vi "SpectrumBinning_NoGraph.vi"(3 "XScale.Maximum":dbl, 4 "BinType":T1, 5 "BinWidth":dbl=1.0, 7 "Enable":bool=TRUE, 8 "error in (no error)":errorcluster, 9 "Signal":dbl[](array[numeric]), 10 "m/z Array":dbl[](array[numeric]), 11 "XScale.Minimum":dbl) -> (0 "error out":errorcluster, 1 "Spectrum":dbl[](array[numeric]), 2 "m/z Array":dbl[](array[numeric]))   [LabVIEW 2013]
uses:
  BinType.ctl
  <vilib>/Analysis/baseanly.llb/Mean (DBL).vi
  <vilib>/Analysis/NI_AALBase.lvlib
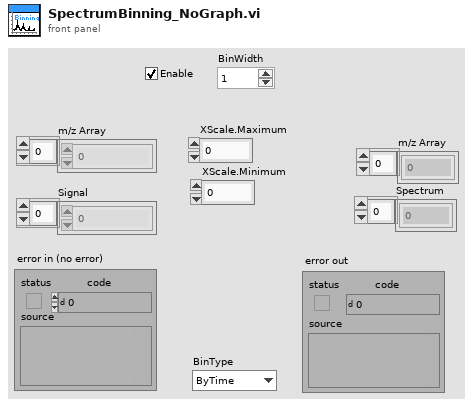
[diagram p1: front panel]
types:
  T1 = typedef "BinType.ctl" = enum16{"ByTime", "ByScreen", "ByMass", "ToUnitMass"}
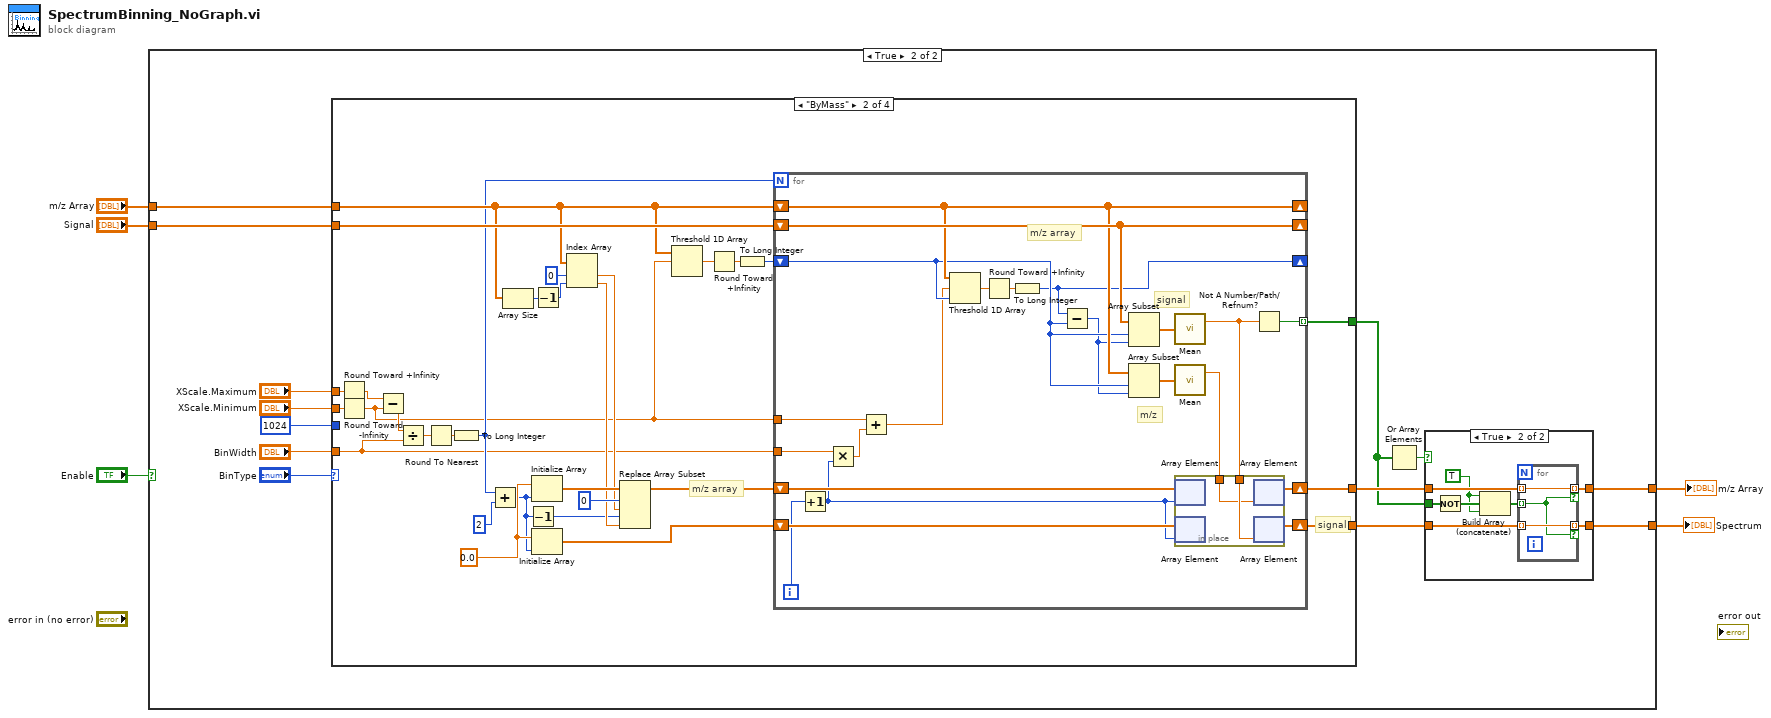
[diagram p0: block diagram]
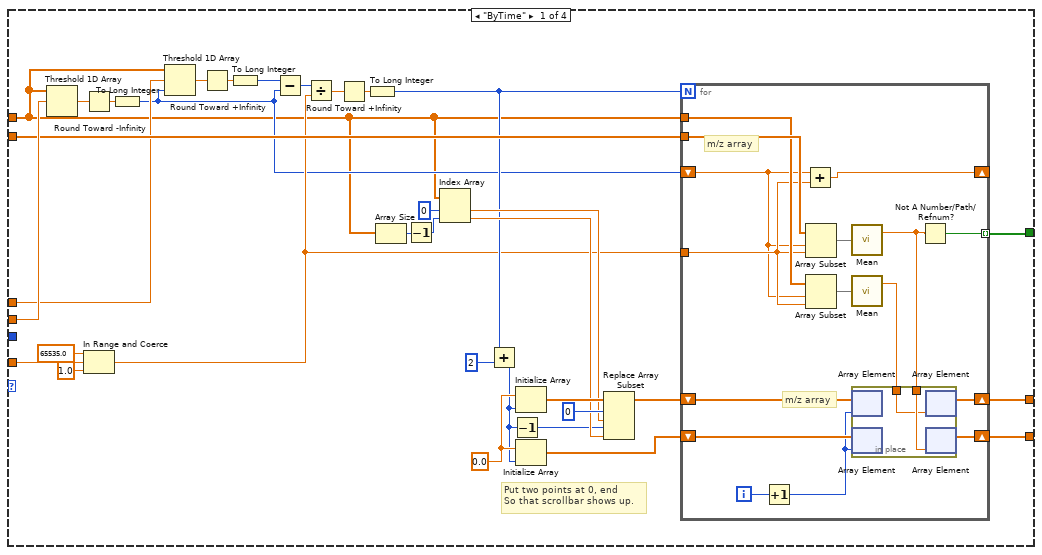
[diagram p4: hidden frame]
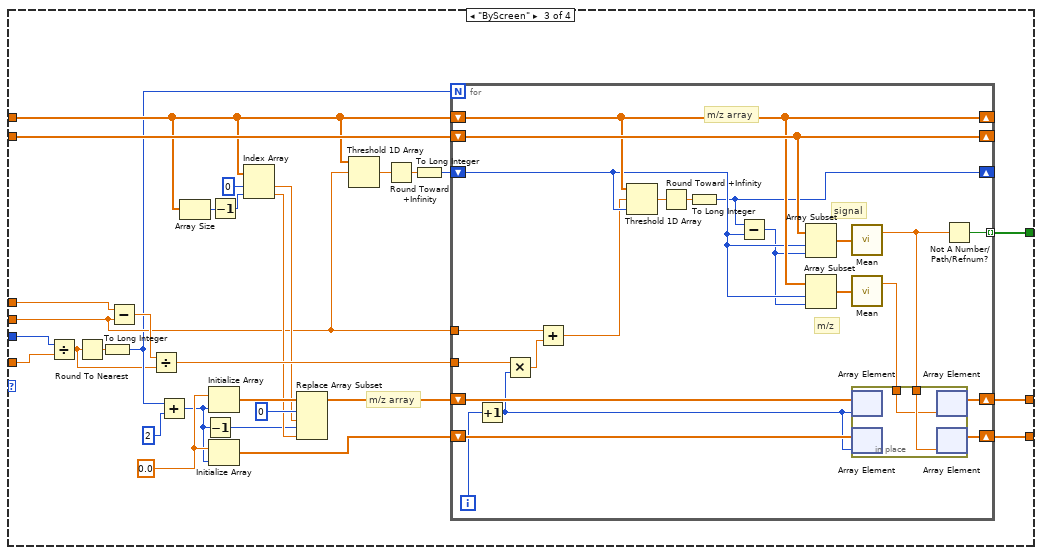
[diagram p5: hidden frame]
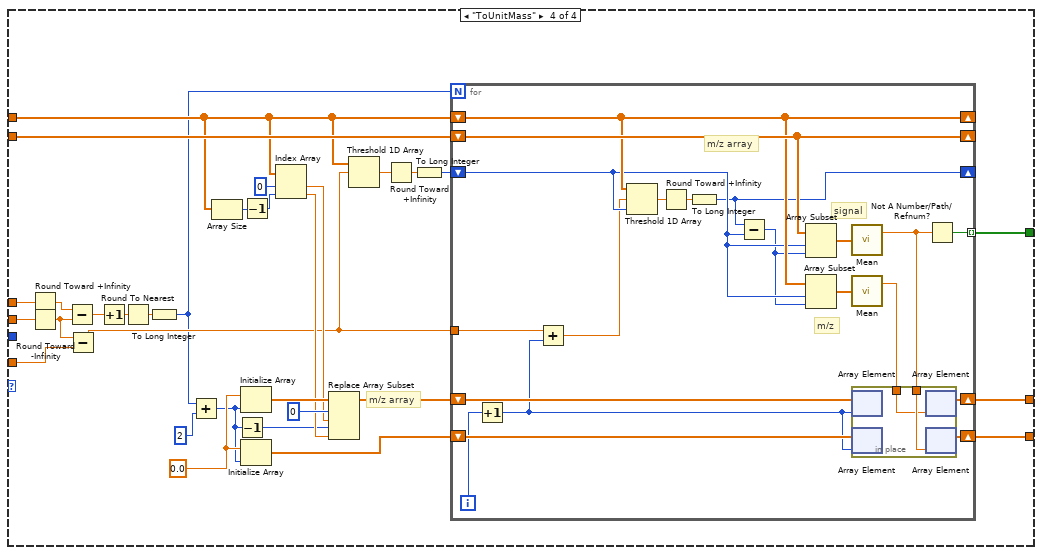
[diagram p6: hidden frame]
diagram:
  n1 = case shown="True" "Enable" {
    tunnel: "Signal" -> [w7 w14]
    tunnel: "m/z Array" -> [w6 w13]
    tunnel: [w6 w9] -> w2
    tunnel: [w7 w8] -> w1
    frame False {
    }
    frame True {
      n2 = case shown="\"ByMass\"" "BinType" {
        tunnel: w14 -> [w53 w115 w169 w224]
        tunnel: w13 -> [w34 w106 w158 w215]
        tunnel: "XScale.Maximum" -> [w38 w100 w152 w209]
        tunnel: "XScale.Minimum" -> [w54 w96 w148 w205]
        tunnel: u32 1024 ("Width") -> [_ _ w145 _]
        tunnel: "BinWidth" -> [w48 w92 w144 w197]
        tunnel: [w40 w87 w141 w195] -> w17
        tunnel: [w41 w86 w142 w196] -> w16
        tunnel: [w39 w88 w140 w194] -> w15
        frame "ByTime" {
          w65 = 0.0 ("x/y")
          # "Put two points at 0, end\nSo that scrollbar shows up."
          n3 = Threshold 1D Array(2:w54, 3:w34) -> (0:w67:dbl)  [unwired: 1 in]
          n4 = Round Toward -Infinity(1:w67) -> (0:w66:dbl)
          n5 = In Range and Coerce(upper limit=65535.0, x=w48, lower limit=1.0) -> (coerced(x)=w44:dbl)  [unwired: 1 out]
          n6 = To Long Integer(number=w66) -> (32bit integer=w37:i32)
          n7 = Threshold 1D Array(1:w37, 2:w38, 3:w34) -> (0:w51:dbl)
          n8 = Round Toward +Infinity(x=w51) -> (ceil(x): smallest int >= x=w52:dbl)
          n9 = To Long Integer(number=w52) -> (32bit integer=w50:i32)
          n10 = Subtract(x=w50, y=w37) -> (x-y=w49:i32)
          n11 = Divide(x=w49, y=w44) -> (x/y=w46:dbl)
          n12 = Round Toward +Infinity(x=w46) -> (ceil(x): smallest int >= x=w47:dbl)
          n13 = To Long Integer(number=w47) -> (32bit integer=w45:i32)
          n14 = Array Size(array=w34) -> (size(s)=w57:i32)
          n15 = Decrement(x=w57) -> (x-1=w55:i32)
          n16 = Index Array(array=w34, index #1=0 ("index"), index #2=w55) -> (element #1=w59:dbl, element #2=w58:dbl)
          n17 = Add(x=w45, y=2) -> (x+y=w36:i32)
          n18 = Decrement(x=w36) -> (x-1=w56:i32)
          n19 = Initialize Array(w65, w36) -> (w64:dbl[])
          n20 = Initialize Array(w65, w36) -> (w63:dbl[])
          n21 = Replace Array Subset(array=w64, new element #1=w59, index #1=0 ("index"), new element #2=w58, index #2=w56) -> (w61:dbl[])
          n22 = for {
            N: w45 -> [_]
            shift-right: [w74] -> _
            shift-left: w37 -> [w72]
            shift-right: [w77] -> w41
            shift-left: w61 -> [w79]
            shift-right: [w76] -> w40
            shift-left: w63 -> [w78]
            tunnel: w44 -> [w73]
            tunnel: [w68] -> w39 mode=indexing
            tunnel: w34 -> [w80]
            tunnel: w53 -> [w83]
            i -> [w71]
            # "m/z array"
            # "m/z array"
            n23 = Increment(x=w71) -> (x+1=w70:i32)
            n24 = Add(x=w72, y=w73) -> (x+y=w74:dbl)
            n25 = Array Subset(array=w83, index=w72, length=w73) -> (w82:dbl[])
            n26 = Array Subset(array=w80, index=w72, length=w73) -> (w81:dbl[])
            n27 = call-poly <vilib>:"Mean.vi"("X"=w82) -> ("mean"=w69:dbl)  [unwired: 1 out]
            n28 = call-poly <vilib>:"Mean.vi"("X"=w81) -> ("mean"=w75:dbl)  [unwired: 1 out]
            n29 = in-place {
              in-place-border: w69 -> [w85]
              in-place-border: w75 -> [w84]
              n30 = in-place-array #1(w79, w70) -> ()  [unwired: 1 out]
              n31 = in-place-array #2(w78, w70) -> ()  [unwired: 1 out]
              n32 = in-place-array #1(w84) -> (w77:dbl[])  [unwired: 1 out]
              n33 = in-place-array #2(w85) -> (w76:dbl[])  [unwired: 1 out]
            }
            n34 = Not A Number/Path/Refnum?(number/path/refnum=w69) -> (NaN/Path/Refnum?=w68:bool)
          }
        }
        frame "ByMass" {
          w111 = 0.0 ("x/y")
          # "signal"
          # "m/z array"
          n35 = Round Toward +Infinity(x=w100) -> (ceil(x): smallest int >= x=w89:dbl)
          n36 = Round Toward -Infinity(1:w96) -> (0:w90:dbl)
          n37 = Subtract(x=w89, y=w90) -> (x-y=w91:dbl)
          n38 = Divide(x=w91, y=w92) -> (x/y=w93:dbl)
          n39 = Round To Nearest(number=w93) -> (nearest integer value=w95:dbl)
          n40 = To Long Integer(number=w95) -> (32bit integer=w94:i32)
          n41 = Add(x=w94, y=2 ("x")) -> (x+y=w99:i32)
          n42 = Array Size(array=w106) -> (size(s)=w101:i32)
          n43 = Decrement(x=w99) -> (x-1=w98:i32)
          n44 = Initialize Array(w111, w99) -> (w110:dbl[])
          n45 = Initialize Array(w111, w99) -> (w109:dbl[])
          n46 = Decrement(x=w101) -> (x-1=w97:i32)
          n47 = Index Array(array=w106, index #1=0 ("index"), index #2=w97) -> (element #1=w103:dbl, element #2=w102:dbl)
          n48 = Replace Array Subset(array=w110, new element #1=w103, index #1=0 ("index"), new element #2=w102, index #2=w98) -> (w105:dbl[])
          n49 = Threshold 1D Array(2:w90, 3:w106) -> (0:w114:dbl)  [unwired: 1 in]
          n50 = Round Toward +Infinity(x=w114) -> (ceil(x): smallest int >= x=w113:dbl)
          n51 = To Long Integer(number=w113) -> (32bit integer=w112:i32)
          n52 = for {
            N: w94 -> [_]
            shift-right: [w137] -> _
            shift-left: w115 -> [w137]
            shift-right: [w134] -> _
            shift-left: w106 -> [w134]
            shift-right: [w123] -> _
            shift-left: w112 -> [w131]
            tunnel: w92 -> [w119]
            shift-right: [w126] -> w86
            shift-left: w105 -> [w129]
            shift-right: [w125] -> w87
            shift-left: w109 -> [w128]
            tunnel: w90 -> [w120]
            tunnel: [w116] -> w88 mode=indexing
            i -> [w127]
            # "signal"
            # "m/z"
            # "m/z array"
            n53 = Increment(x=w127) -> (x+1=w122:i32)
            n54 = Multiply(x=w119, y=w122) -> (x*y=w121:dbl)
            n55 = Add(x=w120, y=w121) -> (x+y=w124:dbl)
            n56 = Threshold 1D Array(1:w131, 2:w124, 3:w134) -> (0:w132:dbl)
            n57 = Round Toward +Infinity(x=w132) -> (ceil(x): smallest int >= x=w133:dbl)
            n58 = To Long Integer(number=w133) -> (32bit integer=w123:i32)
            n59 = Subtract(x=w123, y=w131) -> (x-y=w130:i32)
            n60 = Array Subset(array=w137, index=w131, length=w130) -> (w136:dbl[])
            n61 = Array Subset(array=w134, index=w131, length=w130) -> (w135:dbl[])
            n62 = call-poly <vilib>:"Mean.vi"("X"=w136) -> ("mean"=w117:dbl)  [unwired: 1 out]
            n63 = call-poly <vilib>:"Mean.vi"("X"=w135) -> ("mean"=w118:dbl)  [unwired: 1 out]
            n64 = in-place {
              in-place-border: w117 -> [w139]
              in-place-border: w118 -> [w138]
              n65 = in-place-array #3(w129, w122) -> ()  [unwired: 1 out]
              n66 = in-place-array #4(w128, w122) -> ()  [unwired: 1 out]
              n67 = in-place-array #3(w138) -> (w126:dbl[])  [unwired: 1 out]
              n68 = in-place-array #4(w139) -> (w125:dbl[])  [unwired: 1 out]
            }
            n69 = Not A Number/Path/Refnum?(number/path/refnum=w117) -> (NaN/Path/Refnum?=w116:bool)
          }
        }
        frame "ByScreen" {
          w163 = 0.0 ("x/y")
          # "m/z array"
          n70 = Divide(x=w145, y=w144) -> (x/y=w143:dbl)
          n71 = Round To Nearest(number=w143) -> (nearest integer value=w147:dbl)
          n72 = To Long Integer(number=w147) -> (32bit integer=w146:i32)
          n73 = Subtract(x=w152, y=w148) -> (x-y=w167:dbl)
          n74 = Divide(x=w167, y=w143) -> (x/y=w164:dbl)
          n75 = Add(x=w146, y=2 ("x")) -> (x+y=w151:i32)
          n76 = Array Size(array=w158) -> (size(s)=w153:i32)
          n77 = Decrement(x=w151) -> (x-1=w150:i32)
          n78 = Initialize Array(w163, w151) -> (w162:dbl[])
          n79 = Initialize Array(w163, w151) -> (w161:dbl[])
          n80 = Decrement(x=w153) -> (x-1=w149:i32)
          n81 = Index Array(array=w158, index #1=0 ("index"), index #2=w149) -> (element #1=w155:dbl, element #2=w154:dbl)
          n82 = Replace Array Subset(array=w162, new element #1=w155, index #1=0 ("index"), new element #2=w154, index #2=w150) -> (w157:dbl[])
          n83 = Threshold 1D Array(2:w148, 3:w158) -> (0:w168:dbl)  [unwired: 1 in]
          n84 = Round Toward +Infinity(x=w168) -> (ceil(x): smallest int >= x=w166:dbl)
          n85 = To Long Integer(number=w166) -> (32bit integer=w165:i32)
          n86 = for {
            N: w146 -> [_]
            shift-right: [w191] -> _
            shift-left: w169 -> [w191]
            shift-right: [w188] -> _
            shift-left: w158 -> [w188]
            shift-right: [w177] -> _
            shift-left: w165 -> [w185]
            tunnel: w164 -> [w173]
            shift-right: [w180] -> w142
            shift-left: w157 -> [w183]
            shift-right: [w179] -> w141
            shift-left: w161 -> [w182]
            tunnel: w148 -> [w174]
            tunnel: [w170] -> w140 mode=indexing
            i -> [w181]
            # "signal"
            # "m/z"
            # "m/z array"
            n87 = Increment(x=w181) -> (x+1=w176:i32)
            n88 = Multiply(x=w173, y=w176) -> (x*y=w175:dbl)
            n89 = Add(x=w174, y=w175) -> (x+y=w178:dbl)
            n90 = Threshold 1D Array(1:w185, 2:w178, 3:w188) -> (0:w186:dbl)
            n91 = Round Toward +Infinity(x=w186) -> (ceil(x): smallest int >= x=w187:dbl)
            n92 = To Long Integer(number=w187) -> (32bit integer=w177:i32)
            n93 = Subtract(x=w177, y=w185) -> (x-y=w184:i32)
            n94 = Array Subset(array=w191, index=w185, length=w184) -> (w190:dbl[])
            n95 = Array Subset(array=w188, index=w185, length=w184) -> (w189:dbl[])
            n96 = call-poly <vilib>:"Mean.vi"("X"=w190) -> ("mean"=w171:dbl)  [unwired: 1 out]
            n97 = call-poly <vilib>:"Mean.vi"("X"=w189) -> ("mean"=w172:dbl)  [unwired: 1 out]
            n98 = in-place {
              in-place-border: w171 -> [w193]
              in-place-border: w172 -> [w192]
              n99 = in-place-array #5(w183, w176) -> ()  [unwired: 1 out]
              n100 = in-place-array #6(w182, w176) -> ()  [unwired: 1 out]
              n101 = in-place-array #5(w192) -> (w180:dbl[])  [unwired: 1 out]
              n102 = in-place-array #6(w193) -> (w179:dbl[])  [unwired: 1 out]
            }
            n103 = Not A Number/Path/Refnum?(number/path/refnum=w171) -> (NaN/Path/Refnum?=w170:bool)
          }
        }
        frame "ToUnitMass" {
          w220 = 0.0 ("x/y")
          # "m/z array"
          n104 = Round Toward +Infinity(x=w209) -> (ceil(x): smallest int >= x=w203:dbl)
          n105 = Round Toward -Infinity(1:w205) -> (0:w204:dbl)
          n106 = Subtract(x=w203, y=w204) -> (x-y=w202:dbl)
          n107 = Subtract(x=w204, y=w197) -> (x-y=w200:dbl)
          n108 = Increment(x=w202) -> (x+1=w201:dbl)
          n109 = Round To Nearest(number=w201) -> (nearest integer value=w199:dbl)
          n110 = To Long Integer(number=w199) -> (32bit integer=w198:i32)
          n111 = Add(x=w198, y=2 ("x")) -> (x+y=w208:i32)
          n112 = Array Size(array=w215) -> (size(s)=w210:i32)
          n113 = Decrement(x=w208) -> (x-1=w207:i32)
          n114 = Initialize Array(w220, w208) -> (w219:dbl[])
          n115 = Initialize Array(w220, w208) -> (w218:dbl[])
          n116 = Decrement(x=w210) -> (x-1=w206:i32)
          n117 = Index Array(array=w215, index #1=0 ("index"), index #2=w206) -> (element #1=w212:dbl, element #2=w211:dbl)
          n118 = Replace Array Subset(array=w219, new element #1=w212, index #1=0 ("index"), new element #2=w211, index #2=w207) -> (w214:dbl[])
          n119 = Threshold 1D Array(2:w200, 3:w215) -> (0:w223:dbl)  [unwired: 1 in]
          n120 = Round Toward +Infinity(x=w223) -> (ceil(x): smallest int >= x=w222:dbl)
          n121 = To Long Integer(number=w222) -> (32bit integer=w221:i32)
          n122 = for {
            N: w198 -> [_]
            shift-right: [w244] -> _
            shift-left: w224 -> [w244]
            shift-right: [w241] -> _
            shift-left: w215 -> [w241]
            shift-right: [w230] -> _
            shift-left: w221 -> [w238]
            shift-right: [w233] -> w196
            shift-left: w214 -> [w236]
            shift-right: [w232] -> w195
            shift-left: w218 -> [w235]
            tunnel: w200 -> [w229]
            tunnel: [w225] -> w194 mode=indexing
            i -> [w234]
            # "signal"
            # "m/z"
            # "m/z array"
            n123 = Increment(x=w234) -> (x+1=w227:i32)
            n124 = Add(x=w229, y=w227) -> (x+y=w231:dbl)
            n125 = Threshold 1D Array(1:w238, 2:w231, 3:w241) -> (0:w239:dbl)
            n126 = Round Toward +Infinity(x=w239) -> (ceil(x): smallest int >= x=w240:dbl)
            n127 = To Long Integer(number=w240) -> (32bit integer=w230:i32)
            n128 = Subtract(x=w230, y=w238) -> (x-y=w237:i32)
            n129 = Array Subset(array=w244, index=w238, length=w237) -> (w243:dbl[])
            n130 = Array Subset(array=w241, index=w238, length=w237) -> (w242:dbl[])
            n131 = call-poly <vilib>:"Mean.vi"("X"=w243) -> ("mean"=w226:dbl)  [unwired: 1 out]
            n132 = call-poly <vilib>:"Mean.vi"("X"=w242) -> ("mean"=w228:dbl)  [unwired: 1 out]
            n133 = in-place {
              in-place-border: w226 -> [w246]
              in-place-border: w228 -> [w245]
              n134 = in-place-array #7(w236, w227) -> ()  [unwired: 1 out]
              n135 = in-place-array #8(w235, w227) -> ()  [unwired: 1 out]
              n136 = in-place-array #7(w245) -> (w233:dbl[])  [unwired: 1 out]
              n137 = in-place-array #8(w246) -> (w232:dbl[])  [unwired: 1 out]
            }
            n138 = Not A Number/Path/Refnum?(number/path/refnum=w226) -> (NaN/Path/Refnum?=w225:bool)
          }
        }
      }
      n139 = Or Array Elements(Boolean array=w15) -> (logical OR=w18:bool)
      n140 = case shown="True" w18 {
        tunnel: [w22 w30] -> w9
        tunnel: w16 -> [w22 w29]
        tunnel: [w21 w28] -> w8
        tunnel: w17 -> [w21 w27]
        tunnel: w15 -> [_ w26]
        frame False {
        }
        frame True {
          w23 = TRUE
          n141 = Not(x=w26) -> (.not. x?=w24:bool[])
          n142 = Build Array (concatenate)(w23, w24, w23) -> (w25:bool[])
          n143 = for {
            tunnel: [w33] -> w30 mode=indexing if=w31
            tunnel: w29 -> [w33] mode=indexing
            tunnel: [w32] -> w28 mode=indexing if=w31
            tunnel: w27 -> [w32] mode=indexing
            tunnel: w25 -> [w31] mode=indexing
          }
        }
      }
    }
  }
  "m/z Array" <- w2
  "Spectrum" <- w1
